vi "Unpack Value Change.vi"(11 "VariantValueMsg in":refnum<class "ValueChangeMsg.lvclass">) -> (2 "Value":variant, 3 "Name":string)   [LabVIEW 2015, in "ActorAutoRegistration.lvlib" / "ValueChangeMsg.lvclass"]
uses:
  ValueChangeMsg.lvclass
  ValueChangeMsg.lvclass/ValueChangeMsg.ctl
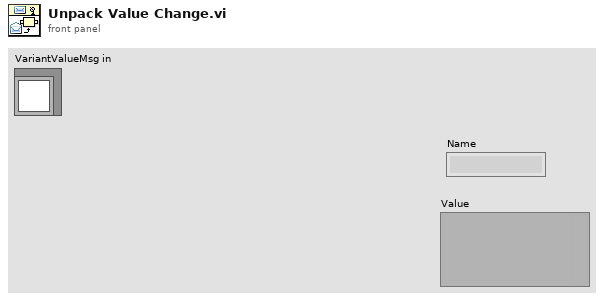
[diagram p1: front panel]
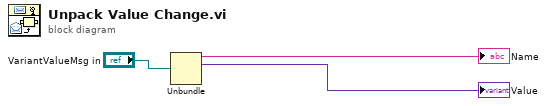
[diagram p0: block diagram]
diagram:
  n1 = Unbundle("VariantValueMsg in") -> (→"Name":string, →"Value":variant)  [unwired: 2 out]
